vi "Write to Property Bag.vi"(8 "error in (no error)":errorcluster, 9 "Prototype in":variant, 10 "Node":string, 11 "CI Deserializer in":refnum<class "CI Deserializer.lvclass">) -> (0 "error out":errorcluster, 1 "Data out":variant, 3 "CI Deserializer out":refnum<class "CI Deserializer.lvclass">)   [LabVIEW 2014, in "CI Deserializer.lvclass"]
uses:
  CI Deserializer.lvclass
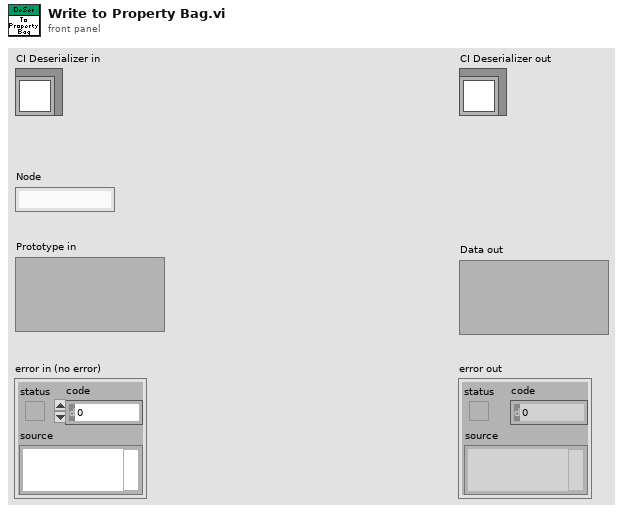
[diagram p1: front panel]
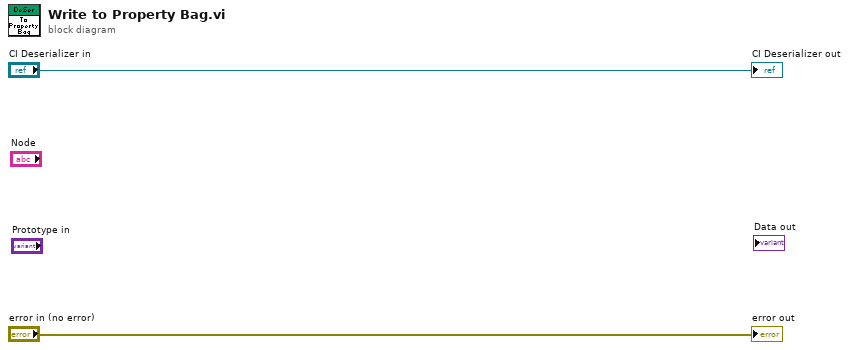
[diagram p0: block diagram]
diagram:
  "error out" <- "error in (no error)"
  "CI Deserializer out" <- "CI Deserializer in"
